vi "mxwScript_API_XMLOption_AutoDiagramChange.vi"(8 "error in (no error)":errorcluster, 10 "auto diagram change?":bool=TRUE, 11 "options in":T1[](array[typedef])) -> (0 "error out":errorcluster, 3 "options out":T1[](array[typedef]))   [LabVIEW 2020]
uses:
  codeGenAPISupport.llb/cgAPI_mxwScript_OptionData.ctl
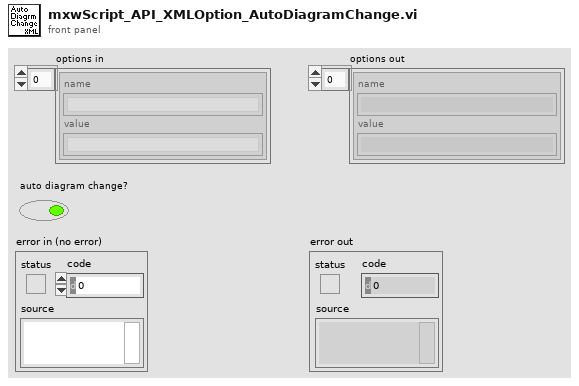
[diagram p1: front panel]
types:
  T1 = typedef "cgAPI_mxwScript_OptionData.ctl" = cluster{"name":string, "value":string}
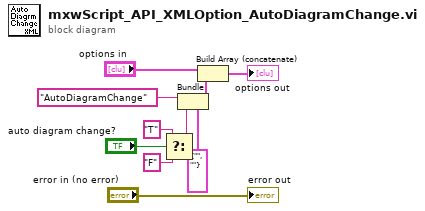
[diagram p0: block diagram]
diagram:
  n1 = Select(t="T", s="auto diagram change?", f="F") -> (s? t:f=w6:string)
  n2 = Bundle(cluster=T1 {"name"="", "value"=""} ("options"), "name"="AutoDiagramChange", "value"=w6) -> (w4:T1)
  n3 = Build Array (concatenate)("options in", w4) -> (→"options out":T1[])
  "error out" <- "error in (no error)"
